vi "Set Panel Color.vi"(0 "VI in":refnum<vi>, 7 "Pane Color":u32, 11 "error in (no error)":errorcluster) -> (15 "error out":errorcluster)   [LabVIEW 2020]
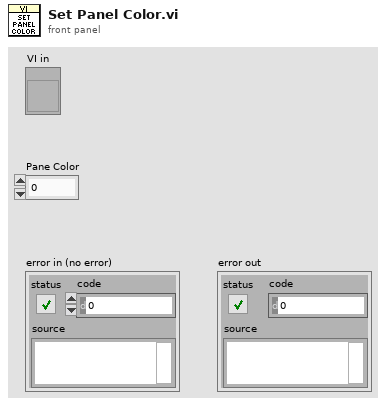
[diagram p1: front panel]
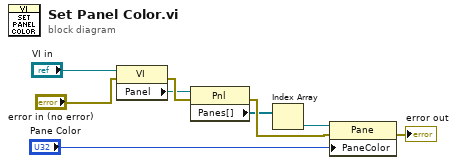
[diagram p0: block diagram]
diagram:
  n1 = property class="VI"(reference="VI in", error in="error in (no error)") -> (error out=w7:errorcluster, "Panel"=w2:refnum<vi>)  [unwired: 1 out]
  n2 = property class="Pnl"(reference=w2, error in=w7) -> (error out=w8:errorcluster, "Panes[]"=w3:refnum<vi>[])  [unwired: 1 out]
  n3 = Index Array(array=w3) -> (element=w4:refnum<vi>)  [unwired: 1 in]
  n4 = property class="Pane"(reference=w4, error in=w8, "PaneColor"="Pane Color") -> (error out=→"error out":errorcluster)  [unwired: 1 out]
